vi "PositionControlTest.vi"() -> ()   [LabVIEW 2009, in "Test.lvlib"]
uses:
  Test.lvlib
  Drive/Drive_ControlMode.ctl
  Drive/Drive_PositionControlMode.ctl
  CAN/SubVIs/CAN Jaguar Control Mode.ctl
  FPGA.lvlib
  Motor.lvlib
  Drive.lvlib
  OWNCAN.lvlib
  CAN.lvlib
panel:
  out "state out":T1
  in  "Maximum Output Voltage":dbl=5.0
  in  "ControlMode":T2
  out "error out":errorcluster
  in  "Type":u8
  in  "Speed limit":dbl=0.5
  in  "Y rel (Right)":dbl
  in  "X rel (Left)":dbl
  in  "stop":bool
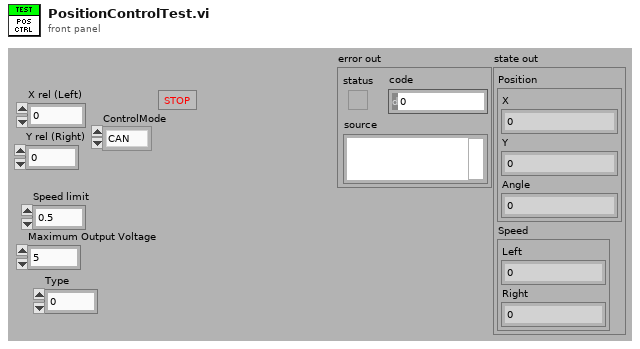
[diagram p1: front panel]
types:
  T1 = cluster{"Position":cluster{"X":dbl, "Y":dbl, "Angle":dbl}, "Speed":cluster{"Left":dbl, "Right":dbl}}
  T2 = typedef "Drive.lvlib/Drive_ControlMode.ctl" = enum16{"CAN", "PWM"}
  T3 = typedef "Drive.lvlib/Drive_PositionControlMode.ctl" = enum16{"TurnThenStraight"}
  T4 = typedef "CAN.lvlib/CAN Jaguar Control Mode.ctl" = enum16{"Percent VBus", "Speed", "Position", "Current"}
  T5 = typedef "OWNCAN.lvlib/CAN Jaguars Ref.ctl" = cluster{"CAN Jaguar Ref Left":T6, "CAN Jaguar Ref Right":T6}
  T6 = typedef "CAN.lvlib/CAN Jaguar Ref.ctl" = cluster{"Device Number":u8, "Control Mode":T4, "Inverted":bool, "Semaphore":T7, "Max Vout":dbl, "DevStatus":errorcluster}
  T7 = typedef "Semaphore RefNum" = refnum<k1>
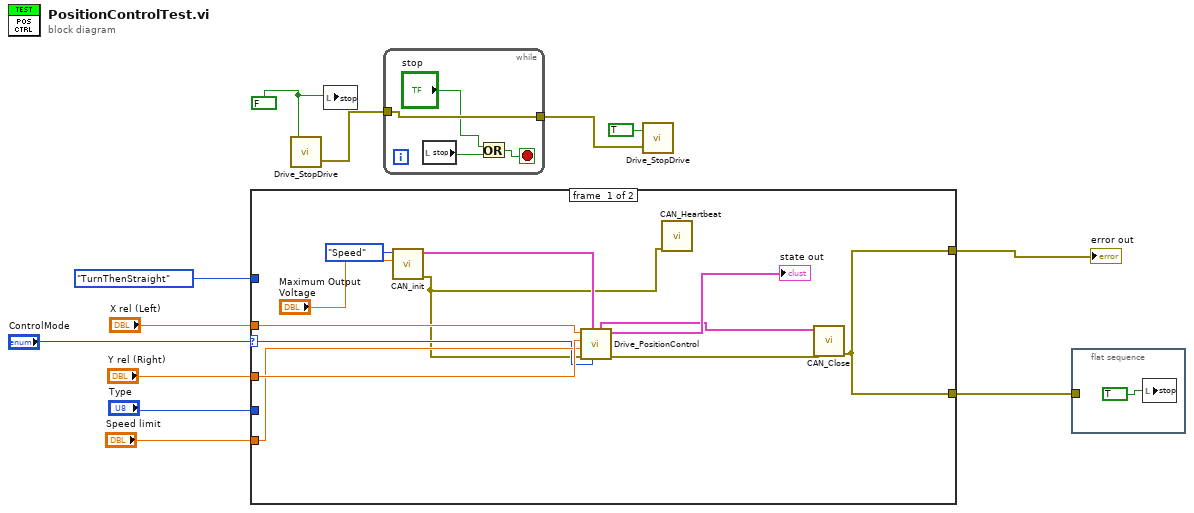
[diagram p0: block diagram]
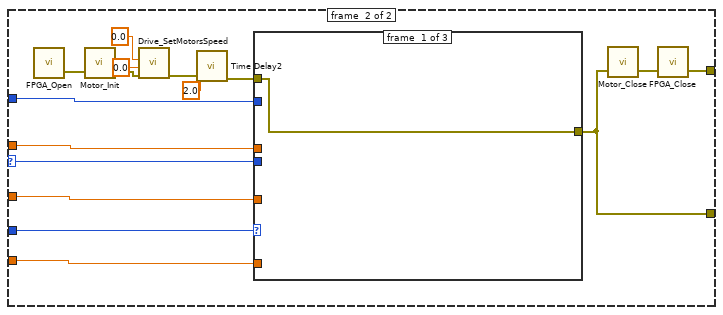
[diagram p2: hidden frame]
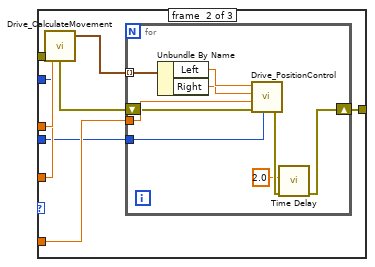
[diagram p3: hidden frame]
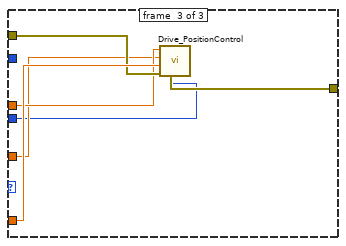
[diagram p4: hidden frame]
diagram:
  w5 = FALSE ("Abort?")
  n1 = case shown="\"CAN\", Default" "ControlMode" {
    selector: "ControlMode" -> [w21 w25]
    tunnel: "X rel (Left)" -> [w24 w39]
    tunnel: "Y rel (Right)" -> [w23 w38]
    tunnel: Drive_PositionControlMode."TurnThenStraight" ("Mode") -> [_ w37]
    tunnel: "Speed limit" -> [w22 w36]
    tunnel: [w14 w35] -> w6
    tunnel: "Type" -> [_ w27]
    tunnel: [w14 w26] -> w2
    frame #0 {
      n2 = call "CAN_init.vi"("Maximum Output Voltage"="Maximum Output Voltage", "Control Mode"=CAN_Jaguar_Control_Mode."Speed") -> ("error out"=w13:errorcluster, "CAN Jaguars Ref"=w20:T5)  [unwired: 6 in]
      n3 = call "Drive_PositionControl.vi"("ControlMode"=w21, "CAN Jaguars Ref"=w20, "error in"=w13, "Speed limit"=w22, "Right_Distance"=w23, "Left_Distance"=w24) -> ("error out"=w15:errorcluster, "state out"=→"state out":T1, "CAN Jaguars Ref out"=w16:T5)  [unwired: 3 in]
      n4 = call "CAN_Heartbeat.vi"("error in"=w13) -> ()  [unwired: 10 in, 1 out]
      n5 = call "CAN_Close.vi"("error in"=w15, "CAN Jaguars Ref"=w16) -> ("error out"=w14:errorcluster)  [unwired: 9 in]
    }
    frame #1 {
      n6 = call "FPGA_Open.vi"() -> ("error out"=w34:errorcluster)  [unwired: 3 in]
      n7 = call "Motor_Init.vi"("error in"=w34) -> ("error out"=w31:errorcluster)  [unwired: 2 in]
      n8 = call "Drive_SetMotorsSpeed.vi"("error in"=w31, "Right_Speed"=0.0, "Left_Speed"=0.0) -> ("error out"=w30:errorcluster)  [unwired: 7 in, 1 out]
      n9 = call "Time Delay2"("error in (no error)"=w30, "Delay Time (s)"=2.0) -> ("error out"=w33:errorcluster)  [unwired: 9 in]
      n10 = case shown="1" w27 {
        tunnel: w39 -> [_ w50 w62]
        tunnel: w38 -> [_ w49 w61]
        tunnel: w37 -> [_ w48 _]
        tunnel: w36 -> [_ w45 w65]
        tunnel: [w41 w44 w63] -> w35
        tunnel: w33 -> [w41 w43 w64]
        tunnel: w25 -> [_ w42 w60]
        frame #0 {
        }
        frame #1 {
          n11 = call "Drive_CalculateMovement.vi"("error in"=w43, "Mode"=w48, "Y rel"=w49, "X rel"=w50) -> ("error out"=w46:errorcluster, "Movements"=w47:cluster{"Left":dbl, "Right":dbl}[])  [unwired: 1 in]
          n12 = for {
            tunnel: w47 -> [w58] mode=indexing
            tunnel: w45 -> [w59]
            shift-right: [w53] -> w44
            shift-left: w46 -> [w55]
            tunnel: w42 -> [w51]
            n13 = Unbundle By Name(w58) -> ("Left"=w57:dbl, "Right"=w56:dbl)
            n14 = call "Drive_PositionControl.vi"("ControlMode"=w51, "error in"=w55, "Speed limit"=w59, "Right_Distance"=w56, "Left_Distance"=w57) -> ("error out"=w54:errorcluster)  [unwired: 4 in, 2 out]
            n15 = call "Time Delay"("error in (no error)"=w54, "Delay Time (s)"=2.0) -> ("error out"=w53:errorcluster)  [unwired: 9 in]
          }
        }
        frame #2 {
          n16 = call "Drive_PositionControl.vi"("ControlMode"=w60, "error in"=w64, "Speed limit"=w65, "Right_Distance"=w61, "Left_Distance"=w62) -> ("error out"=w63:errorcluster)  [unwired: 4 in, 2 out]
        }
      }
      n17 = call "Motor_Close.vi"("error in"=w35) -> ("error out"=w40:errorcluster)  [unwired: 2 in]
      n18 = call "FPGA_Close.vi"("error in (no error)"=w40) -> ("error out"=w26:errorcluster)  [unwired: 2 in]
    }
  }
  "error out" <- w2
  n19 = call "Drive_StopDrive.vi"("Stop? (T)"=w5) -> ("error out"=w12:errorcluster)  [unwired: 2 in]
  n20 = local write "stop"(w5) -> ()
  n21 = while {
    tunnel: w12 -> [w69]
    tunnel: [w69] -> w11
    stop <- w68 stop-if-true
    n22 = local read "stop"() -> (w67:bool)
    n23 = Or(x="stop", y=w67) -> (x .or. y?=w68:bool)
  }
  n24 = call "Drive_StopDrive.vi"("error in"=w11, "Stop? (T)"=TRUE ("Abort?")) -> ()  [unwired: 1 in, 1 out]
  n25 = flat-sequence {
    tunnel: w6 -> [_]
    frame #0 {
      n26 = local write "stop"(TRUE) -> ()
    }
  }
